vi "CLSUIP_GetUnlockPrompt.vi"(1 "ElementWrapperRetooler":refnum<class "ElementWrapperRetooler.lvclass">) -> (0 "localized prompt 2":string="%s is password-protected.  You must enter the password to create a wrapper VI for this member VI.")   [LabVIEW 2021, in "MemberVICreation.lvlib" / "ElementWrapperRetooler.lvclass"]
uses:
  <resource>/Framework/Providers/LVClassLibrary/NewAccessors/ElementWrapperRetooler/ElementWrapperRetooler.lvclass
panel:
  in  "localized prompt":string="%s is password-protected.  You must enter the password to create a wrapper VI for this member VI."
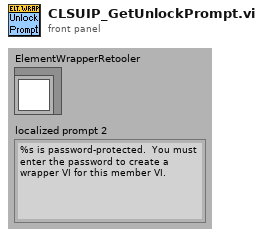
[diagram p1: front panel]
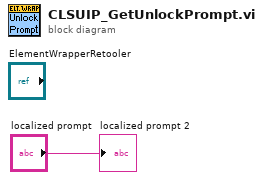
[diagram p0: block diagram]
diagram:
  "localized prompt 2" <- "localized prompt"
